vi "GEN_Speed-coded_overlay.vi"(0 "Speed-coded overlay refnum in":T1, 1 "Speed array in":dbl[](array[numeric]), 5 "Full track array":T2(array[cluster]), 7 "Multiline grouping, samples":i32=100, 9 "Samples full merge, every N":i32=1000, 11 "error in (no error)":errorcluster) -> (4 "Speed-coded overlay refnum out":T1, 15 "error out":errorcluster)   [LabVIEW 2018, in "Tracker.lvlib"]
uses:
  Tracker.lvlib
  <vilib>/vision/Image Controls.llb/IMAQ Image.ctl
  Controls/CTL_Color_ramp.ctl
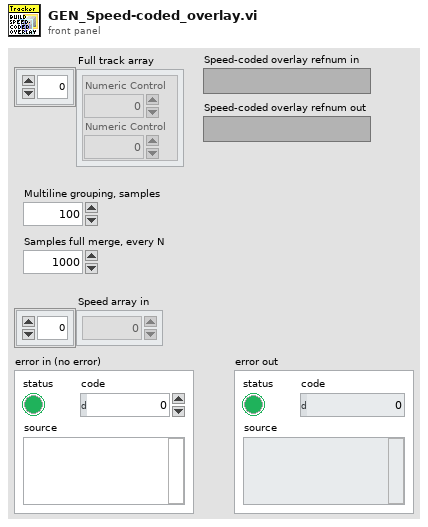
[diagram p1: front panel]
types:
  T1 = typedef "IMAQ Image.ctl" = refnum<image>
  T2 = cluster{"Numeric Control":dbl, "Numeric Control":dbl}[]
  T3 = typedef "Tracker.lvlib/CTL_Color_ramp.ctl" = u32[]
  T4 = cluster{"Numeric Control":dbl, "Numeric Control":dbl}
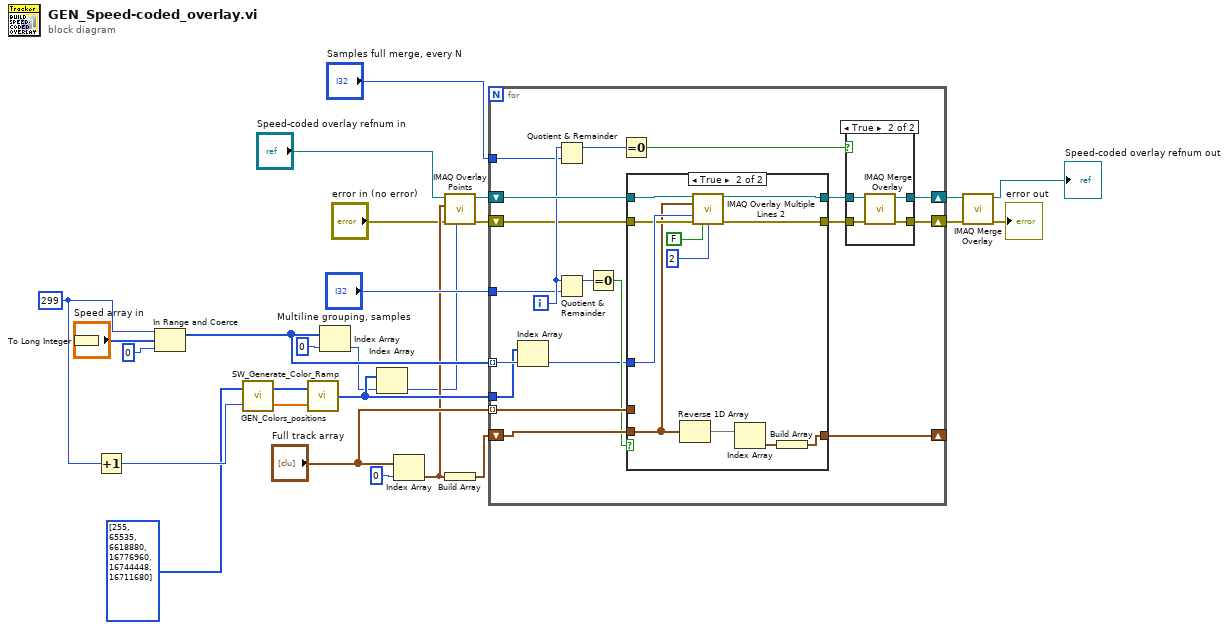
[diagram p0: block diagram]
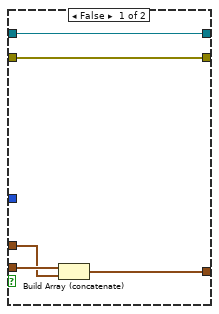
[diagram p2: hidden frame]
diagram:
  w20 = 299
  n1 = To Long Integer(number="Speed array in") -> (32bit integer=w5:i32[])
  n2 = Increment(x=w20) -> (x+1=w19:i32)
  n3 = In Range and Coerce(upper limit=w20, x=w5, lower limit=0) -> (coerced(x)=w17:i32[])  [unwired: 1 out]
  n4 = call "GEN_Colors_positions.vi"("Highest color position"=w19, "Initial colors ramp array in"=T3 [255, 65535, 6618880, 16776960, 16744448, 16711680] ("Initial colors ramp array")) -> ("Colors positions"=w22:dbl[], "Initial colors ramp array out"=w21:T3)
  n5 = call "SW_Generate_Color_Ramp.vi"("Colors rel. pos."=w22, "Colors array"=w21) -> ("Colors array"=w23:u32[])
  n6 = Index Array(array=w17, index=0) -> (element=w10:i32)
  n7 = Index Array(array=w23, index=w10) -> (element=w7:u32)
  n8 = Index Array(array="Full track array", index=0) -> (element=w12:T4)
  n9 = call "IMAQ Overlay Points"("Color"=w7, "error in (no error)"="error in (no error)", "Point"=w12, "Image"="Speed-coded overlay refnum in") -> ("error out"=w1:errorcluster, "Image Out"=w11:T1)  [unwired: 6 in]
  n10 = Build Array(w12) -> (w13:T2)
  n11 = for {
    shift-right: [w45] -> w14
    shift-left: w11 -> [w40]
    tunnel: "Full track array" -> [w43] mode=indexing
    shift-right: [w31] -> w15
    shift-left: w1 -> [w34]
    shift-right: [w39] -> _
    shift-left: w13 -> [w42]
    tunnel: "Multiline grouping, samples" -> [w35]
    tunnel: "Samples full merge, every N" -> [w33]
    tunnel: w17 -> [w30] mode=indexing
    tunnel: w23 -> [w29]
    i -> [w36]
    n12 = Index Array(array=w29, index=w30) -> (element=w28:u32)
    n13 = Quotient & Remainder(x=w36, y=w33) -> (x-y*floor(x/y)=w44:i32)  [unwired: 1 out]
    n14 = Quotient & Remainder(x=w36, y=w35) -> (x-y*floor(x/y)=w38:i32)  [unwired: 1 out]
    n15 = Equal To 0?(x=w38) -> (x = 0?=w37:bool)
    n16 = Equal To 0?(x=w44) -> (x = 0?=w46:bool)
    n17 = case shown="True" w37 {
      tunnel: w43 -> [w48 _]
      tunnel: w42 -> [w50 w56]
      tunnel: w28 -> [_ w62]
      tunnel: w34 -> [w47 w61]
      tunnel: [w51 w60] -> w41
      tunnel: [w47 w59] -> w32
      tunnel: w40 -> [w51 w58]
      tunnel: [w49 w53] -> w39
      frame False {
        n18 = Build Array (concatenate)(w50, w48) -> (w49:T2)
      }
      frame True {
        n19 = Reverse 1D Array(array=w56) -> (reversed array=w55:T2)
        n20 = call "IMAQ Overlay Multiple Lines 2"("Image"=w58, "Line End Points"=w56, "Color"=w62, "error in (no error)"=w61, "Maintain Width?"=FALSE, "Width"=u32 2) -> ("Image Out"=w60:T1, "error out"=w59:errorcluster)  [unwired: 8 in]
        n21 = Index Array(array=w55) -> (element=w54:T4)  [unwired: 1 in]
        n22 = Build Array(w54) -> (w53:T2)
      }
    }
    n23 = case shown="True" w46 {
      tunnel: w41 -> [w64 w68]
      tunnel: [w64 w67] -> w45
      tunnel: w32 -> [w63 w66]
      tunnel: [w63 w65] -> w31
      frame False {
      }
      frame True {
        n24 = call "IMAQ Merge Overlay"("error in (no error)"=w66, "Image Src"=w68) -> ("error out"=w65:errorcluster, "Image Dst Out"=w67:T1)  [unwired: 8 in]
      }
    }
  }
  n25 = call "IMAQ Merge Overlay"("error in (no error)"=w15, "Image Src"=w14) -> ("error out"=→"error out":errorcluster, "Image Dst Out"=→"Speed-coded overlay refnum out":T1)  [unwired: 8 in]
